vi "3 OCU.vi"() -> ()   [LabVIEW 2011]
doc: "This is the current implementation of the operator control unit (OCU) for small RC boat controlled by a host computer. The following features are currently implemented:\n- override control of the rudden angle and sail value by control interface or using keys\n- ability to add missions before and during a run\n- indicators for all relevant system status information\n\nAuthor: Jared Kirschner"
uses:
  2-RIO/2 Typedefs/setpoints to boat.ctl
  2-RIO/2 Typedefs/sail setpt.ctl
  2-RIO/2 Typedefs/rudder angle.ctl
  2-RIO/2 Typedefs/Velocity.ctl
  2-RIO/2 Typedefs/apparent wind direction.ctl
  2-RIO/2 Typedefs/apparent wind speed.ctl
  2-RIO/2 Typedefs/apparent wind.ctl
  2-RIO/2 Typedefs/heading.ctl
  2-RIO/2 Typedefs/UTM Location.ctl
  2-RIO/2 Typedefs/Which Boat.ctl
  2-RIO/2 Typedefs/generalized sensor status.ctl
  2-RIO/2 Typedefs/indicator LED.ctl
  2-RIO/2 Typedefs/generalized actuator status.ctl
  2x3-RIO-OCU Comm/2x3 Typedefs/ocuWaypoints.ctl
  2x3-RIO-OCU Comm/2x3 Typedefs/ocuWaypoint.ctl
  2x3-RIO-OCU Comm/2x3 Typedefs/waypointTypes.ctl
  2-RIO/2 Typedefs/manual override.ctl
  2-RIO/2 Globals/2 Global.vi
panel:
  out "Override Rudder Angle":dbl(slide) scale=-30.0..30.0
  out "Override Sail Value":dbl(slide) scale=0.0..1.0
  in  "OVERRIDE?":bool
  in  "OCU Tab Control":T1(tab)
  out "Connected":bool
  in  "Connect":bool
  out "Rudder Actuator Status":T2
  out "Sail Actuator Status":T2
  out "Wind Sensor Status":T4
  out "Location Sensor Status":T4
  out "Direction Sensor Status":T4
  in  "Load":bool
  in  "Load Mission":path
  in  "Globals":T5(tab)
  out "Which Boat Am I?":T6
  in  "Battery Voltage":dbl
  out "Robot\nHeading":T7 format="%05.1f"
  out "Robot UTM Location":T8
  out "Robot Velocity":T9
  out "Overview Image":T10(plugin-control)
  out "Absolute Wind":T9
  out "Apparent Wind\nDirection":T11
  out "Apparent Wind\nSpeed":T12
  out "Apparent Wind":T13
  out "List of Waypoints":T14 {"Waypoints Array"."Point Type" items=["Drive", "Round Port", "Round Starboard", "Stay"]}
  out "Setpoints to boat":T17
  out "Sail Position":T18
  out "Rudder Angle":T19
  in  "Waypoint":T15 {"Point Type" items=["Drive", "Round Port", "Round Starboard", "Stay"]}
  in  "Add Waypoint":bool
  # "Manual Overide Control"
  # "Full Out = RIGHT"
  # "Out = UP"
  # "In = DOWN"
  # "Full In = LEFT"
  # "PORT"
  # "STARB"
  # "A"
  # "G"
  # "S"
  # "<--"
  # "D"
  # "-->"
  # "F"
  # "should be a map here that you can clique on"
  # "As Measured"
  # "From Planning Functions"
  # "Path Planning"
  # "(this is not a cluster because subitems\nare generated in parallel code)"
  # "Mission Definition Stuff Goes HERE"
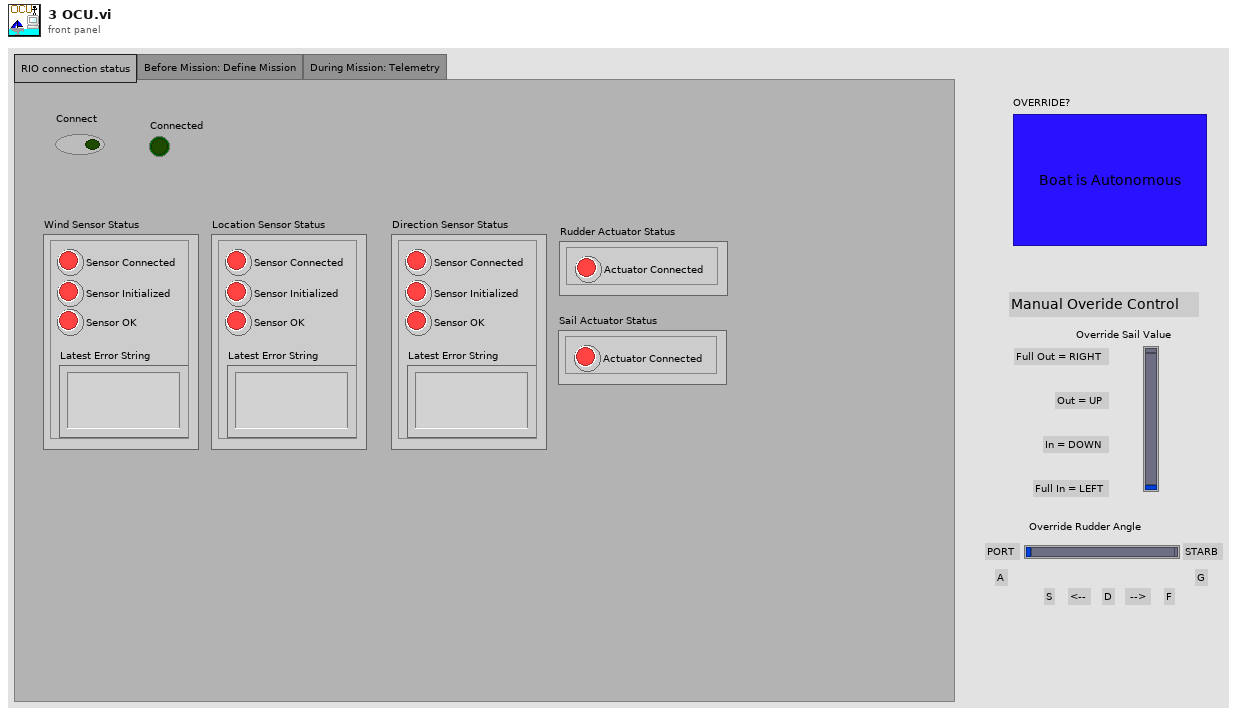
[diagram p1: front panel]
types:
  T1 = enum32{"RIO connection status", "Before Mission: Define Mission", "During Mission: Telemetry"}
  T2 = typedef "generalized actuator status.ctl" = cluster{"Actuator Connected":T3}
  T3 = typedef "indicator LED.ctl" = bool
  T4 = typedef "generalized sensor status.ctl" = cluster{"Sensor Connected":T3, "Sensor Initialized":T3, "Sensor OK":T3, "Latest Error String":string}
  T5 = enum32{"How Am I", "Where Am I", "What's Around Me", "Path Planning"}
  T6 = typedef "Which Boat.ctl" = enum16{"Competition Boat", "Small RC", "Simulation"}
  T7 = typedef "heading.ctl" = dbl
  T8 = typedef "UTM Location.ctl" = cluster{"UTM Zone":dbl, "Hemisphere":enum16{"North", "South"}, "East":dbl, "North":dbl}
  T9 = typedef "Velocity.ctl" = cluster{"East":dbl, "North":dbl}
  T10 = typedef "IMAQ Image.ctl" = refnum<image>
  T11 = typedef "apparent wind direction.ctl" = dbl
  T12 = typedef "apparent wind speed.ctl" = dbl
  T13 = typedef "apparent wind.ctl" = cluster{"Toward Fore":dbl, "Toward Starboard":dbl}
  T14 = typedef "ocuWaypoints.ctl" = cluster{"Waypoints Array":T15[], "Current Waypoint":dbl}
  T15 = typedef "ocuWaypoint.ctl" = cluster{"Point Type":T16, "Dist/Time":dbl, "UTM Location":T8}
  T16 = typedef "waypointTypes.ctl" = u16
  T17 = typedef "setpoints to boat.ctl" = cluster{"Sail Position":T18, "Rudder Angle":T19}
  T18 = typedef "sail setpt.ctl" = dbl
  T19 = typedef "rudder angle.ctl" = dbl
  T20 = typedef "manual override.ctl" = cluster{"Override Active":bool, "Setpoints":T17}
  T21 = typedef "eventvkey.ctl" = enum16{"ASCII", "Enter", "Return", "Shift", "Ctrl", "Alt", "Cmd", "Opt", "Caps", "NumLock", "Clear", "Break", "Up", "Down", "Left", "Right", "Insert", "Delete", "Home", "End", "PageUp", "PageDown", "Escape", "Help", "Pause", "ScrollLock", "F1", "F2", "F3", "F4", "F5", "F6", "F7", "F8", "F9", "F10", "F11", "F12", "F13", "F14", "F15", "F16", "F17", "F18", "F19", "F20", "F21", "F22", "F23", "F24", "Play", "VolumeUp", "VolumeDown", "Mute", "Two Byte Char"}
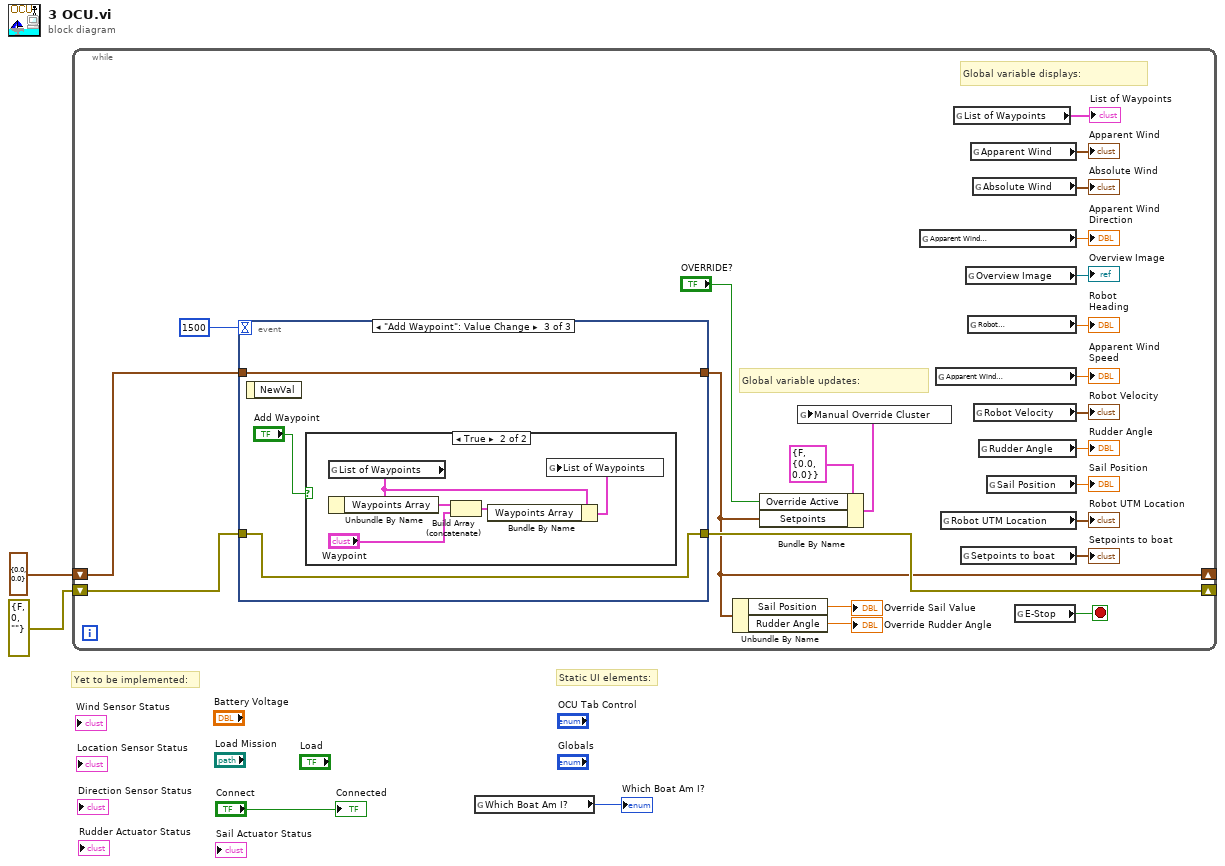
[diagram p0: block diagram]
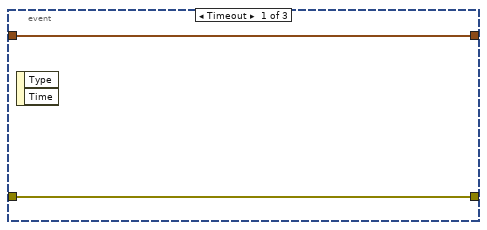
[diagram p2: hidden frame]
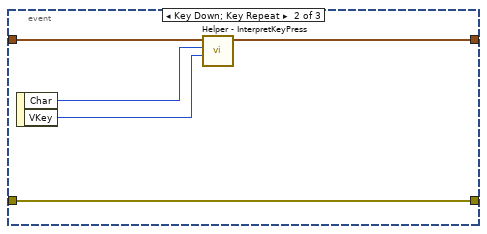
[diagram p3: hidden frame]
diagram:
  # "Static UI elements:"
  # "Yet to be implemented:"
  n1 = while {
    shift-right: [w10] -> _
    shift-left: errorcluster {"status"=FALSE, "code"=0, "source"=""} ("error out") -> [w11]
    shift-right: [w8] -> _
    shift-left: T17 {"Sail Position"=0.0, "Rudder Angle"=0.0} ("Setpoints") -> [w15]
    stop <- w27 stop-if-true
    # "Global variable updates:"
    # "Global variable displays:"
    n2 = event shown="[2] \"Add Waypoint\": Value Change" {
      selector: _ -> [_ _ _]
      dyn-events: _ -> [_ _ _]
      timeout: 1500 -> [_ _ _]
      tunnel: w15 -> [w29 w34 w37]
      tunnel: [w29 w33 w37] -> w8
      tunnel: w11 -> [w28 w30 w36]
      tunnel: [w28 w30 w36] -> w10
      event Timeout {
        n3 = event-data() -> ()  [unwired: 1 in, 2 out]
      }
      event Key Down; Key Repeat {
        n4 = event-data() -> ("Char"=w32:i16, "VKey"=w31:T21)  [unwired: 1 in]
        n5 = call "Helper - InterpretKeyPress.vi"("VKey"=w31, "Char"=w32, "Command In"=w34) -> ("Command Out"=w33:T17)  [unwired: 8 in]
      }
      event "Add Waypoint": Value Change {
        n6 = event-data() -> ()  [unwired: 1 in, 1 out]
        n7 = case shown="True" "Add Waypoint" {
          frame False {
          }
          frame True {
            n8 = global read "2 Global.vi" "List of Waypoints"() -> (w40:T14)
            n9 = Unbundle By Name(w40) -> ("Waypoints Array"=w42:T15[])
            n10 = Build Array (concatenate)(w42, "Waypoint") -> (w39:T15[])
            n11 = Bundle By Name(cluster=w40, "Waypoints Array"=w39) -> (w38:T14)
            n12 = global write "2 Global.vi" "List of Waypoints"(w38) -> ()
          }
        }
      }
    }
    n13 = Unbundle By Name(w8) -> ("Sail Position"=→"Override Sail Value":T18, "Rudder Angle"=→"Override Rudder Angle":T19)
    n14 = Bundle By Name(cluster=T20 {"Override Active"=FALSE, "Setpoints"={"Sail Position"=0.0, "Rudder Angle"=0.0}} ("Manual Override Cluster"), "Override Active"="OVERRIDE?", "Setpoints"=w8) -> (w12:T20)
    n15 = global write "2 Global.vi" "Manual Override Cluster"(w12) -> ()
    n16 = global read "2 Global.vi" "Apparent Wind\nDirection"() -> (→"Apparent Wind\nDirection":T11)
    n17 = global read "2 Global.vi" "Apparent Wind\nSpeed"() -> (→"Apparent Wind\nSpeed":T12)
    n18 = global read "2 Global.vi" "Robot UTM Location"() -> (→"Robot UTM Location":T8)
    n19 = global read "2 Global.vi" "List of Waypoints"() -> (→"List of Waypoints":T14)
    n20 = global read "2 Global.vi" "Setpoints to boat"() -> (→"Setpoints to boat":T17)
    n21 = global read "2 Global.vi" "Overview Image"() -> (→"Overview Image":T10)
    n22 = global read "2 Global.vi" "Robot\nHeading"() -> (→"Robot\nHeading":T7)
    n23 = global read "2 Global.vi" "Apparent Wind"() -> (→"Apparent Wind":T13)
    n24 = global read "2 Global.vi" "Absolute Wind"() -> (→"Absolute Wind":T9)
    n25 = global read "2 Global.vi" "Robot Velocity"() -> (→"Robot Velocity":T9)
    n26 = global read "2 Global.vi" "Rudder Angle"() -> (→"Rudder Angle":T19)
    n27 = global read "2 Global.vi" "Sail Position"() -> (→"Sail Position":T18)
    n28 = global read "2 Global.vi" "E-Stop"() -> (w27:bool)
  }
  n29 = global read "2 Global.vi" "Which Boat Am I?"() -> (→"Which Boat Am I?":T6)
  "Connected" <- "Connect"
